vi "SettingsTextTranslator.vi"(3 "Current Settings:":T1={"Requested Genlock"="1.0", "Duration "="0.99847300000000005", "Overclock "="0", "Requested Horizontal "="733.0", "Requested Pretrigger "="50.0", "Requested Duration "="1.0", "Vertical "="816", "Requested Vertical "="831.0", "Reqested Frame Rate "="1000.0", "Frame Rate "="497.76007964161272", "Horizontal "="720", "Exposure "="0.002", "Genlock "="1", "Subsample "="0", "Requested Exposure "="0.002", "Iso "="500", "Requested Overclock"="0.0", "Requested Subsample"="0.0", "Pretrigger"="50.0", "Requested Iso"="500.0", "Multishot"="1.0", "Gain"="1.25"}) -> (1 "Settings":string)   [LabVIEW 2015]
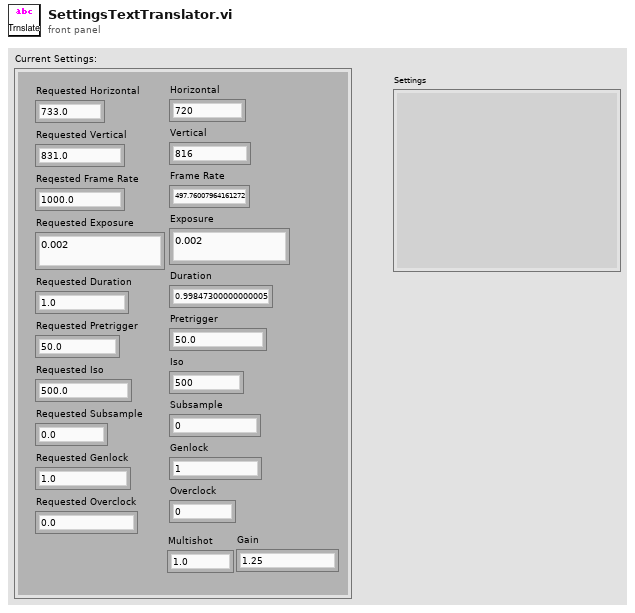
[diagram p1: front panel]
types:
  T1 = cluster{"Requested Genlock":string, "Duration ":string, "Overclock ":string, "Requested Horizontal ":string, "Requested Pretrigger ":string, "Requested Duration ":string, "Vertical ":string, "Requested Vertical ":string, "Reqested Frame Rate ":string, "Frame Rate ":string, "Horizontal ":string, "Exposure ":string, "Genlock ":string, "Subsample ":string, "Requested Exposure ":string, "Iso ":string, "Requested Overclock":string, "Requested Subsample":string, "Pretrigger":string, "Requested Iso":string, "Multishot":string, "Gain":string}
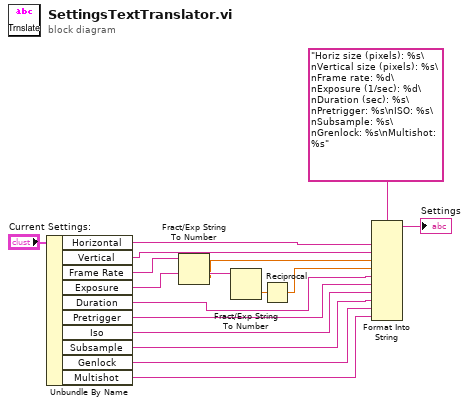
[diagram p0: block diagram]
diagram:
  n1 = Unbundle By Name("Current Settings:") -> ("Horizontal"=w13:string, "Vertical"=w12:string, "Frame Rate"=w11:string, "Exposure"=w10:string, "Duration"=w7:string, "Pretrigger"=w6:string, "Iso"=w5:string, "Subsample"=w4:string, "Genlock"=w3:string, "Multishot"=w2:string)
  n2 = Fract/Exp String To Number(string=w11) -> (number=w1:dbl)  [unwired: 3 in, 1 out]
  n3 = Fract/Exp String To Number(string=w10) -> (number=w9:dbl)  [unwired: 3 in, 1 out]
  n4 = Reciprocal(x=w9) -> (1/x=w8:dbl)
  n5 = Format Into String(format string="Horiz size (pixels): %s\nVertical size (pixels): %s\nFrame rate: %d\nExposure (1/sec): %d\nDuration (sec): %s\nPretrigger: %s\nISO: %s\nSubsample: %s\nGrenlock: %s\nMultishot: %s", w13, w12, w1, w8, w7, w6, w5, w4, w3, w2) -> (resulting string=→"Settings":string)  [unwired: 2 in, 1 out]
